vi "FInal_LAB_Task.vi"() -> ()   [LabVIEW 2020]
panel:
  out "Soil_Moisture":dbl(knob) scale=0.0..100.0
  out "Tank_Level":dbl(slide) scale=0.0..100.0
  in  "VISA resource name":refnum<visa-resource-name>
  in  "Table Control":string[][](table)
  out "Humidity":dbl(knob) scale=0.0..100.0
  out "Temp":dbl(slide) scale=0.0..50.0
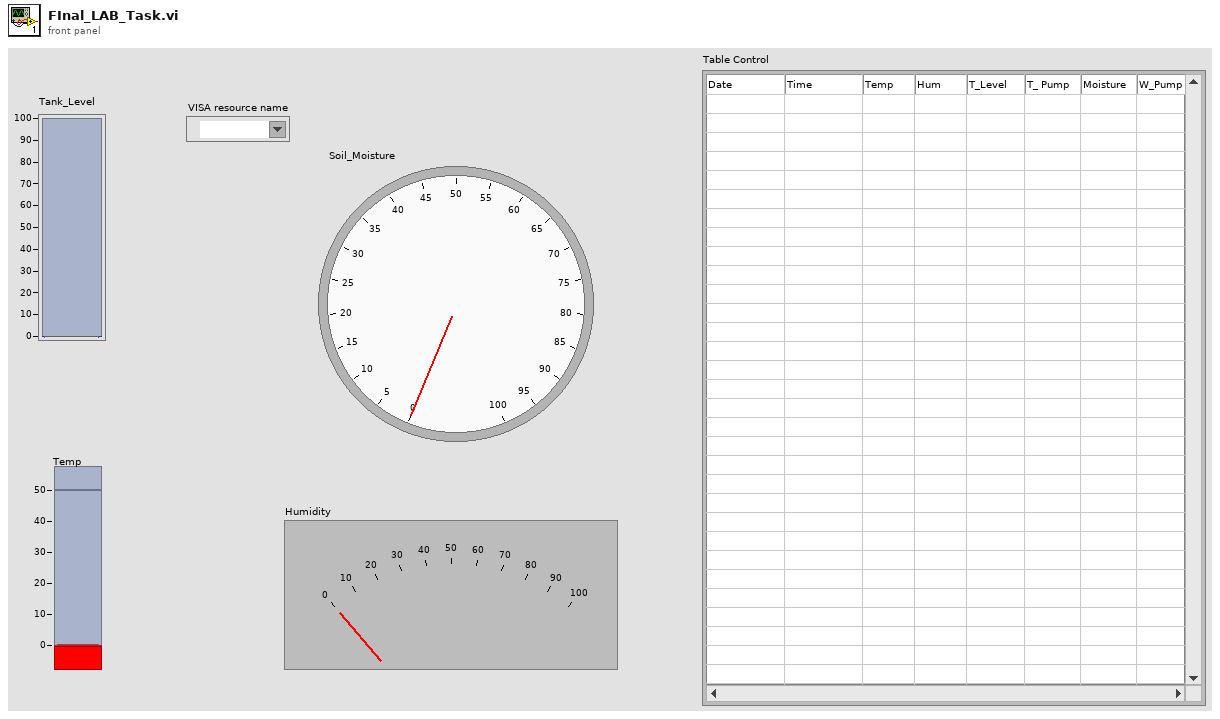
[diagram p1: front panel]
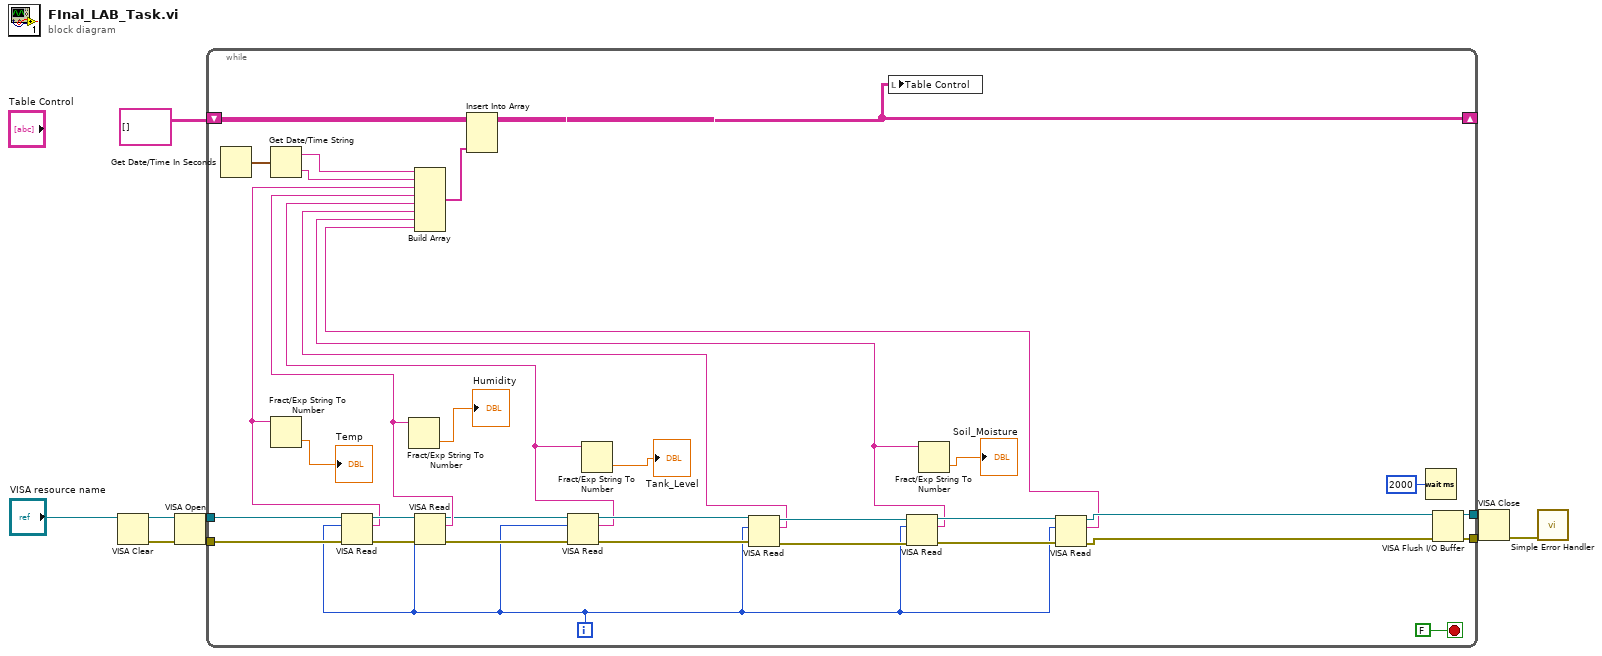
[diagram p0: block diagram]
diagram:
  n1 = VISA Clear(VISA resource name="VISA resource name") -> (VISA resource name out=w8:refnum<visa-resource-name>, error out=w9:errorcluster)  [unwired: 1 in]
  n2 = VISA Open(error in (no error)=w9, VISA resource name=w8) -> (VISA resource name=w6:refnum<visa-resource-name>, error out=w5:errorcluster)  [unwired: 3 in]
  n3 = while {
    tunnel: w6 -> [w44]
    tunnel: w5 -> [w43]
    tunnel: [w40] -> w3
    tunnel: [w39] -> w4
    shift-right: [w36] -> _
    shift-left: string[][] [] -> [w37]
    i -> [w16]
    stop <- FALSE stop-if-true
    n4 = Get Date/Time In Seconds() -> (seconds since 1Jan1904=w33:timestamp)
    n5 = Get Date/Time String(seconds (now)=w33) -> (date string=w32:string, time string=w31:string)  [unwired: 2 in]
    n6 = VISA Read(VISA resource name=w44, byte count=w16, error in (no error)=w43) -> (VISA resource name out=w41:refnum<visa-resource-name>, read buffer=w30:string, error out=w42:errorcluster)  [unwired: 1 out]
    n7 = Fract/Exp String To Number(string=w30) -> (number=→"Temp":dbl)  [unwired: 3 in, 1 out]
    n8 = VISA Read(VISA resource name=w41, byte count=w16, error in (no error)=w42) -> (VISA resource name out=w26:refnum<visa-resource-name>, read buffer=w29:string, error out=w25:errorcluster)  [unwired: 1 out]
    n9 = Fract/Exp String To Number(string=w29) -> (number=→"Humidity":dbl)  [unwired: 3 in, 1 out]
    n10 = VISA Read(VISA resource name=w26, byte count=w16, error in (no error)=w25) -> (VISA resource name out=w24:refnum<visa-resource-name>, read buffer=w14:string, error out=w20:errorcluster)  [unwired: 1 out]
    n11 = Fract/Exp String To Number(string=w14) -> (number=→"Tank_Level":dbl)  [unwired: 3 in, 1 out]
    n12 = VISA Read(VISA resource name=w24, byte count=w16, error in (no error)=w20) -> (VISA resource name out=w23:refnum<visa-resource-name>, read buffer=w10:string, error out=w19:errorcluster)  [unwired: 1 out]
    n13 = VISA Read(VISA resource name=w23, byte count=w16, error in (no error)=w19) -> (VISA resource name out=w22:refnum<visa-resource-name>, read buffer=w12:string, error out=w18:errorcluster)  [unwired: 1 out]
    n14 = Fract/Exp String To Number(string=w12) -> (number=→"Soil_Moisture":dbl)  [unwired: 3 in, 1 out]
    n15 = VISA Read(VISA resource name=w22, byte count=w16, error in (no error)=w18) -> (VISA resource name out=w21:refnum<visa-resource-name>, read buffer=w15:string, error out=w17:errorcluster)  [unwired: 1 out]
    n16 = Build Array(w32, w31, w30, w29, w14, w10, w12, w15) -> (w28:string[])
    n17 = Insert Into Array(array=w37, new element=w28) -> (w36:string[][])  [unwired: 2 in]
    n18 = local write "Table Control"(w36) -> ()
    n19 = Wait (ms)(milliseconds to wait=u32 2000) -> ()  [unwired: 1 out]
    n20 = VISA Flush I/O Buffer(VISA resource name=w21, error in (no error)=w17) -> (VISA resource name out=w39:refnum<visa-resource-name>, error out=w40:errorcluster)  [unwired: 1 in]
  }
  n21 = VISA Close(VISA resource name=w4, error in (no error)=w3) -> (error out=w7:errorcluster)
  n22 = call <vilib>:"Simple Error Handler.vi"("error in (no error)"=w7) -> ()  [unwired: 4 in, 5 out]
